vi "initial magnetic fit parameters.vi"(6 "L/z0":dbl format="%#_13g", 7 "decimation factor":i32=1, 9 "T":dbl, 10 "t0":dbl, 11 "mag no drive":T2[](array[typedef])) -> (0 "fitter error":bool, 3 "initial guess":T1)   [LabVIEW 2017]
uses:
  typedefs/reading.ctl
  typedefs/readingType.ctl
  typedefs/magnetic field fit.ctl
  <vilib>/gmath/NumericalOptimization/Nonlinear Curve Fit LM.vi
  <vilib>/gmath/NumericalOptimization/Nonlinear Curve Fit LM bound.vi
  <vilib>/gmath/NI_Gmath.lvlib
  <vilib>/Analysis/NI_AAL_Geometry.lvlib
  <vilib>/Analysis/NI_AALPro.lvlib
  <vilib>/Analysis/NI_AALBase.lvlib
panel:
  out "phi":dbl[](array[numeric])
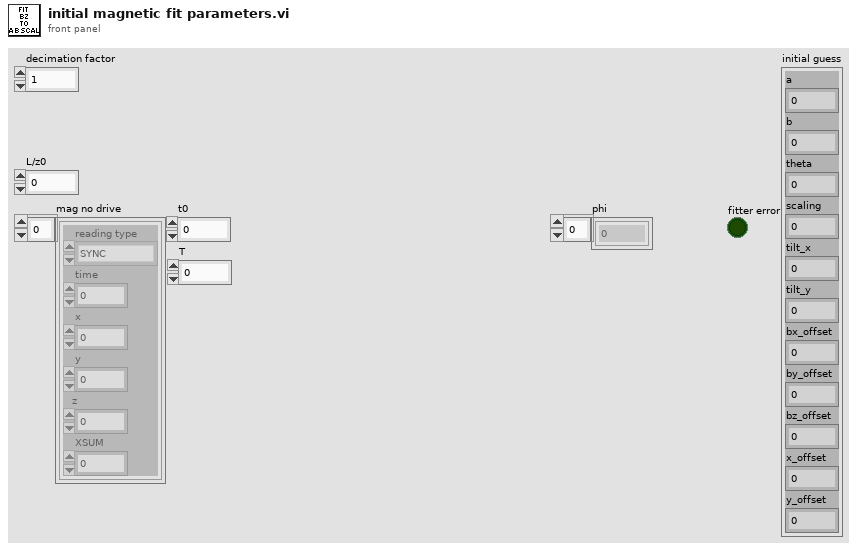
[diagram p1: front panel]
types:
  T1 = typedef "magnetic field fit.ctl" = cluster{"a":dbl, "b":dbl, "theta":dbl, "scaling":dbl, "tilt_x":dbl, "tilt_y":dbl, "bx_offset":dbl, "by_offset":dbl, "bz_offset":dbl, "x_offset":dbl, "y_offset":dbl}
  T2 = typedef "reading.ctl" = cluster{"reading type":T3, "time":fxp<+,48,48>, "x":sgl, "y":sgl, "z":sgl, "XSUM":u8}
  T3 = typedef "readingType.ctl" = enum8{"SYNC", "DETVAL", "COILI", "MAGVEC", "ACCVEC"}
  T4 = cluster{"parameter minimum":dbl[], "parameter maximum":dbl[]}
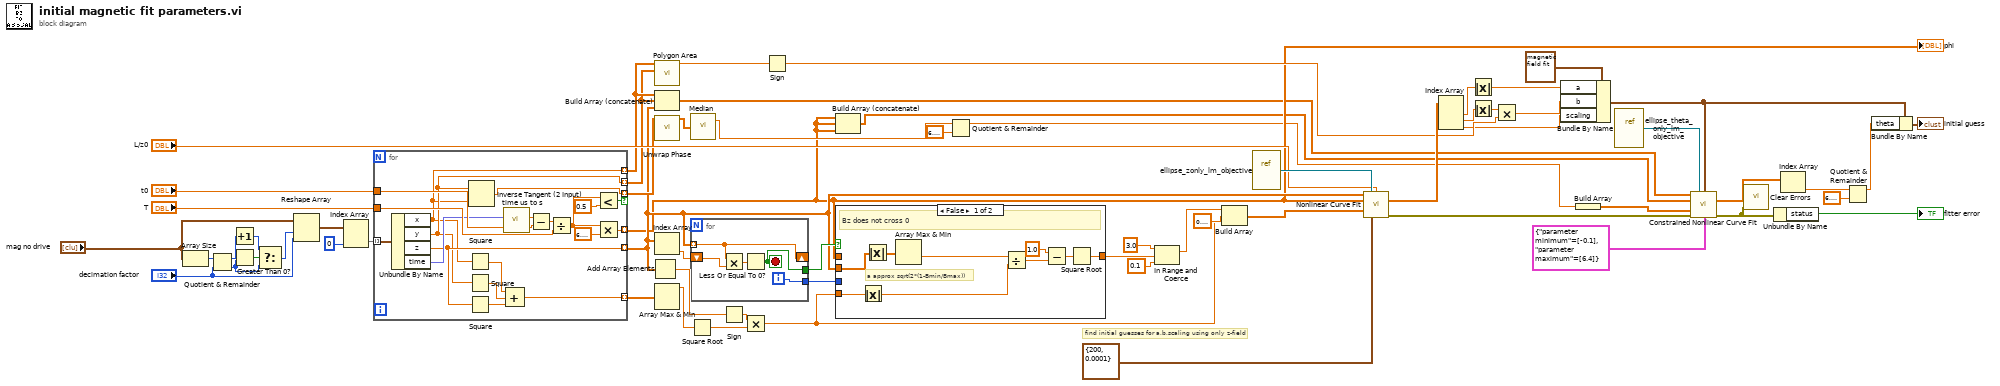
[diagram p0: block diagram]
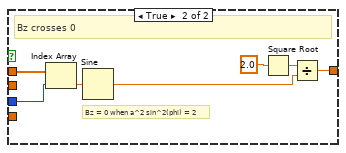
[diagram p2: hidden frame]
diagram:
  # "find initial guesses for a,b,scaling using only z-field"
  n1 = Array Size(array="mag no drive") -> (size(s)=w11:i32)
  n2 = Quotient & Remainder(x=w11, y="decimation factor") -> (x-y*floor(x/y)=w10:i32, floor(x/y)=w7:i32)
  n3 = Increment(x=w7) -> (x+1=w8:i32)
  n4 = Greater Than 0?(x=w10) -> (x > 0?=w9:bool)
  n5 = Select(t=w8, s=w9, f=w7) -> (s? t:f=w5:i32)
  n6 = Reshape Array("mag no drive", w5, "decimation factor") -> (w3:T2[][])
  n7 = Index Array(array=w3, index (col)=0 ("disabled index (col)")) -> (element=w1:T2[])  [unwired: 1 in]
  n8 = for {
    tunnel: w1 -> [w83] mode=indexing
    tunnel: "T" -> [w80]
    tunnel: "t0" -> [w82]
    tunnel: [w77] -> w30 mode=indexing
    tunnel: [w67] -> w33 mode=indexing
    tunnel: [w68] -> w32 mode=indexing
    tunnel: [w76] -> w31 mode=indexing
    tunnel: [w72] -> w44 mode=indexing
    tunnel: [w66] -> w41 mode=indexing if=w65
    n9 = Unbundle By Name(w83) -> ("x"=w67:sgl, "y"=w68:sgl, "z"=w76:sgl, "time"=w78:fxp<+,48,48>)
    n10 = Square(x=w67) -> (x^2=w75:sgl)
    n11 = Square(x=w68) -> (x^2=w74:sgl)
    n12 = Square(x=w76) -> (x^2=w73:sgl)
    n13 = Inverse Tangent (2 Input)(1:w67, 2:w68) -> (0:w66:sgl)
    n14 = call "time us to s.vi"("time (us)"=w78) -> ("time (s)"=w71:dbl)  [unwired: 10 in]
    n15 = Compound Arithmetic op=ADD(w75, w74, w73) -> (w72:sgl)
    n16 = Subtract(x=w71, y=w82) -> (x-y=w81:dbl)
    n17 = Divide(x=w81, y=w80) -> (x/y=w70:dbl)
    n18 = Less?(x=w70, y=0.5) -> (x < y?=w65:bool)
    n19 = Multiply(x=w70, y=6.283185307179586) -> (x*y=w77:dbl)
  }
  "phi" <- w30
  n20 = Add Array Elements(numeric array=w31) -> (sum=w61:sgl)
  n21 = call <vilib>:"Polygon Area.vi"("Y"=w32, "X"=w33) -> ("signed area"=w54:dbl)  [unwired: 8 in, 1 out]
  n22 = Build Array (concatenate)(w33, w32, w31) -> (w28:sgl[])
  n23 = call <vilib>:"Unwrap Phase.vi"("Phase"=w41) -> ("Unwrapped Phase"=w40:dbl[])  [unwired: 9 in, 1 out]
  n24 = Index Array(array=w31) -> (element=w50:sgl)  [unwired: 1 in]
  n25 = Array Max & Min(array=w44) -> (max value=w43:sgl)  [unwired: 3 out]
  n26 = Square Root(x=w43) -> (sqrt(x)=w60:sgl)
  n27 = call <vilib>:"Median.vi"("X"=w40) -> ("median"=w39:dbl)  [unwired: 1 out]
  n28 = for {
    tunnel: w31 -> [w87] mode=indexing
    shift-right: [w87] -> _
    shift-left: w50 -> [w88]
    tunnel: [w85] -> w49
    tunnel: [w84] -> w48
    i -> [w84]
    stop <- w85 stop-if-true
    n29 = Multiply(x=w87, y=w88) -> (x*y=w86:sgl)
    n30 = Less Or Equal To 0?(x=w86) -> (x <= 0?=w85:bool)
  }
  n31 = Sign(1:w61) -> (0:w59:sgl)
  n32 = Multiply(x=w59, y=w60) -> (x*y=w12:sgl)
  n33 = Sign(1:w54) -> (0:w51:dbl)
  n34 = Build Array (concatenate)(w30, w30, w30) -> (w29:dbl[])
  n35 = case shown="False" w49 {
    tunnel: w48 -> [_ w103]
    tunnel: w30 -> [_ w104]
    tunnel: [w93 w98] -> w47
    tunnel: w31 -> [w97 _]
    tunnel: w12 -> [w91 _]
    frame False {
      # "a approx sqrt(2*(1-Bmin/Bmax))"
      # "Bz does not cross 0"
      n36 = Absolute Value(x=w91) -> (abs(x)=w90:sgl)
      n37 = Absolute Value(x=w97) -> (abs(x)=w92:sgl[])
      n38 = Array Max & Min(array=w92) -> (min value=w96:sgl)  [unwired: 3 out]
      n39 = Divide(x=w96, y=w90) -> (x/y=w95:sgl)
      n40 = Subtract(x=1.0, y=w95) -> (x-y=w89:dbl)
      n41 = Square Root(x=w89) -> (sqrt(x)=w93:dbl)
    }
    frame True {
      # "Bz = 0 when a^2 sin^2(phi) = 2"
      # "Bz crosses 0"
      n42 = Index Array(array=w104, index=w103) -> (element=w101:dbl)
      n43 = Sine(x=w101) -> (sin(x)=w100:dbl)
      n44 = Square Root(x=2.0) -> (sqrt(x)=w99:dbl)
      n45 = Divide(x=w99, y=w100) -> (x/y=w98:dbl)
    }
  }
  n46 = Quotient & Remainder(x=w39, y=6.283185307179586) -> (x-y*floor(x/y)=w27:dbl)  [unwired: 1 out]
  n47 = In Range and Coerce(upper limit=3.0, x=w47, lower limit=0.1) -> (coerced(x)=w42:dbl)  [unwired: 1 out]
  n48 = Build Array(w42, sgl 0.1 ("element"), w12) -> (w55:dbl[])
  n49 = vi-ref "ellipse_zonly_lm_objective.vi"() -> (w58:refnum<vi>)
  n50 = call-poly <vilib>:"Nonlinear Curve Fit.vi"("Y"=w31, "f(x,a)"=w58, "data"="L/z0", "X"=w30, "initial parameters"=w55, "termination"=cluster{"max iteration":i32, "tolerance":dbl} {"max iteration"=200, "tolerance"=0.0001}) -> ("best fit parameters"=w53:dbl[], "error out"=w17:errorcluster)  [unwired: 4 in, 4 out]
  n51 = Index Array(array=w53) -> (element #1=w36:dbl, element #2=w52:dbl, element #3=w34:dbl)  [unwired: 3 in]
  n52 = Absolute Value(x=w36) -> (abs(x)=w15:dbl)
  n53 = Absolute Value(x=w52) -> (abs(x)=w14:dbl)
  n54 = Multiply(x=w14, y=w51) -> (x*y=w35:dbl)
  n55 = Bundle By Name(cluster=T1 {"a"=0.0, "b"=0.0, "theta"=0.0, "scaling"=0.0, "tilt_x"=0.0, "tilt_y"=0.0, "bx_offset"=0.0, "by_offset"=0.0, "bz_offset"=0.0, "x_offset"=0.0, "y_offset"=0.0} ("parameters"), "a"=w15, "b"=w35, "scaling"=w34) -> (w20:T1)
  n56 = Build Array(w27) -> (w26:dbl[])
  n57 = vi-ref "ellipse_theta_only_lm_objective.vi"() -> (w21:refnum<vi>)
  n58 = call-poly <vilib>:"Constrained Nonlinear Curve Fit.vi"("Y"=w28, "f(x,a)"=w21, "data"=w20, "X"=w29, "initial parameters"=w26, "error in (no error)"=w17, "parameter bounds"=T4 {"parameter minimum"=[-0.1], "parameter maximum"=[6.4]}) -> ("best fit parameters"=w23:dbl[], "error out"=w16:errorcluster)  [unwired: 3 in, 4 out]
  n59 = call <vilib>:"Clear Errors.vi"("error in (no error)"=w16) -> ()  [unwired: 5 in, 2 out]
  n60 = Unbundle By Name(w16) -> ("status"=→"fitter error":bool)
  n61 = Index Array(array=w23) -> (element=w22:dbl)  [unwired: 1 in]
  n62 = Quotient & Remainder(x=w22, y=6.283185307179586) -> (x-y*floor(x/y)=w19:dbl)  [unwired: 1 out]
  n63 = Bundle By Name(cluster=w20, "theta"=w19) -> (→"initial guess":T1)
